vi "Find Syncronous Frequency.vi"(9 "DDS clock":dbl=125000000.0 format="%_13p", 10 "DDS modulus":i64=15120 format="0x%x (%d)", 11 "Frequency":dbl format="%#_15p") -> (3 "Actual frequency":dbl format="%_19p")   [LabVIEW 2016]
uses:
  <vilib>/gmath/NI_AAL_MathFunc.lvlib
panel:
  out "Array":i64[](array[numeric])
  out "x+y":i64[](array[numeric])
  out "x*y":i64
  out "x/y":i64
  out "Prime Factors":i64[](array[numeric])
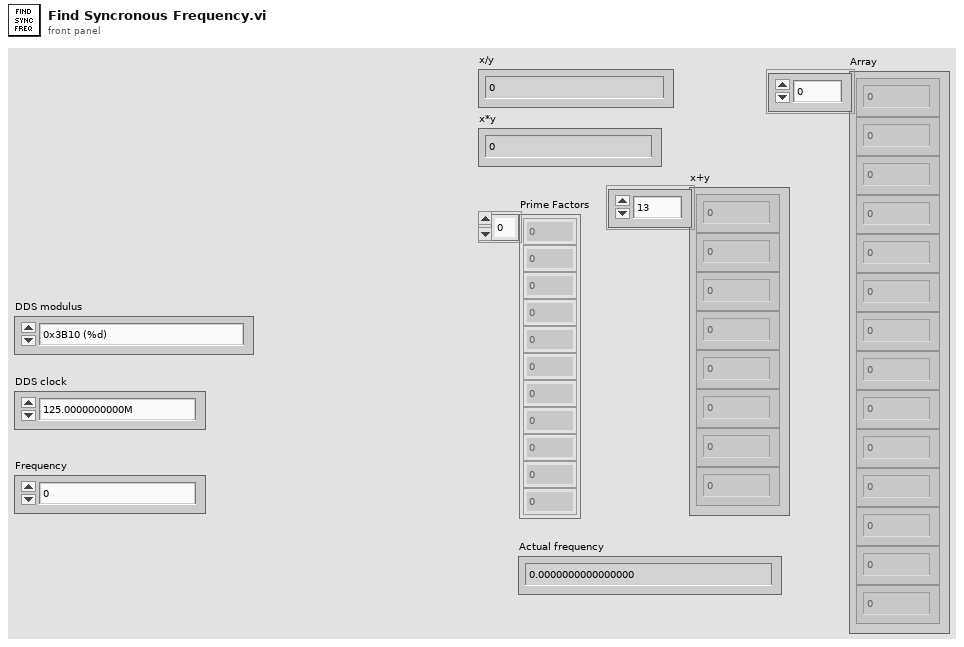
[diagram p1: front panel]
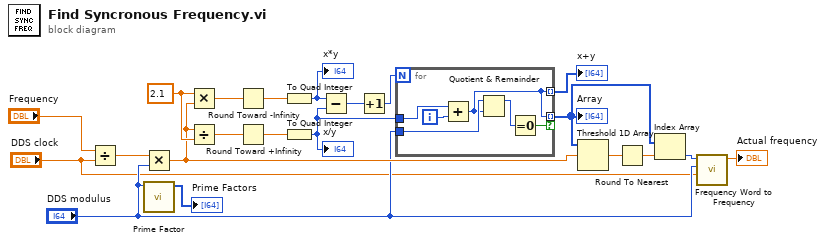
[diagram p0: block diagram]
diagram:
  w20 = 2.1 ("y")
  n1 = Divide(x="Frequency", y="DDS clock") -> (x/y=w18:dbl)
  n2 = Multiply(x=w18, y="DDS modulus") -> (x*y=w9:dbl)
  n3 = call <vilib>:"Prime Factor.vi"("n"="DDS modulus") -> ("Prime Factors"=→"Prime Factors":i64[])  [unwired: 9 in]
  n4 = Multiply(x=w20, y=w9) -> (x*y=w16:dbl)
  n5 = Divide(x=w9, y=w20) -> (x/y=w17:dbl)
  n6 = Round Toward -Infinity(1:w16) -> (0:w15:dbl)
  n7 = Round Toward +Infinity(x=w17) -> (ceil(x): smallest int >= x=w14:dbl)
  n8 = To Quad Integer(1:w15) -> (0:w12:i64)
  "x*y" <- w12
  n9 = To Quad Integer(1:w14) -> (0:w10:i64)
  "x/y" <- w10
  n10 = Subtract(x=w12, y=w10) -> (x-y=w13:i64)
  n11 = Increment(x=w13) -> (x+1=w5:i64)
  n12 = for {
    N: w5 -> [_]
    tunnel: "DDS modulus" -> [w27]
    tunnel: [w22] -> w11 mode=indexing
    tunnel: w10 -> [w26]
    tunnel: [w22] -> w7 mode=indexing if=w23
    i -> [w25]
    n13 = Add(x=w26, y=w25) -> (x+y=w22:i64)
    n14 = Quotient & Remainder(x=w27, y=w22) -> (x-y*floor(x/y)=w24:i64)  [unwired: 1 out]
    n15 = Equal To 0?(x=w24) -> (x = 0?=w23:bool)
  }
  "x+y" <- w11
  "Array" <- w7
  n16 = Threshold 1D Array(2:w9, 3:w7) -> (0:w8:dbl)  [unwired: 1 in]
  n17 = Round To Nearest(number=w8) -> (nearest integer value=w6:dbl)
  n18 = Index Array(array=w7, index=w6) -> (element=w4:i64)
  n19 = call "Frequency Word to Frequency .vi"("DDS clock"="DDS clock", "DDS modulus"="DDS modulus", "Frequency word"=w4) -> ("Frequency"=→"Actual frequency":dbl)  [unwired: 8 in]
